vi "ConvertPB_AOupdates.vi"(0 "PB VLIW Array in":T2(array[cluster]) {"Output Bits" format="%x"}, 1 "Definitions":T1={"External MemorySize"=32768, "Internal Memory Size"=512, "Overhead Ticks"=3, "Min Delay Loops"=3, "Loop Count Correction"=1, "Long Delay Loop Count Correction"=2, "Min Instruction Ticks"=6, "Long Delay Ticks"=4294967295, "Clock Period (s)"=1e-08, "Overhead Time (s)"=3e-08, "Min Instruction Cycle Time (s)"=9e-08, "Long Delay Time (s) "=42.94967298} {"Long Delay Time (s)" format="%.8p"; "Min Instruction Cycle Time (s)" format="%.0p"; "Overhead Time (s)" format="%.0p"; "Clock Period (s)" format="%.0p"; "Long Delay Ticks" format="%.0x"}, 2 "error in (no error)":errorcluster, 3 "Full trigger mask":u32 format="%x") -> (5 "PB VLIW Array out":T2(array[cluster]) {"Output Bits" format="%x"}, 6 "error out":errorcluster)   [LabVIEW 2013, in "PulseBlaster.lvlib"]
doc: "Convert AO updates to two pulses to allow consecutive AO pulses. Replicates the whole PB sequence execpt for channel 22 (AO tigger) and the PB halt channel."
uses:
  PulseBlaster.lvlib
panel:
  # "(Period*Long D Ticks)+Overhead time"
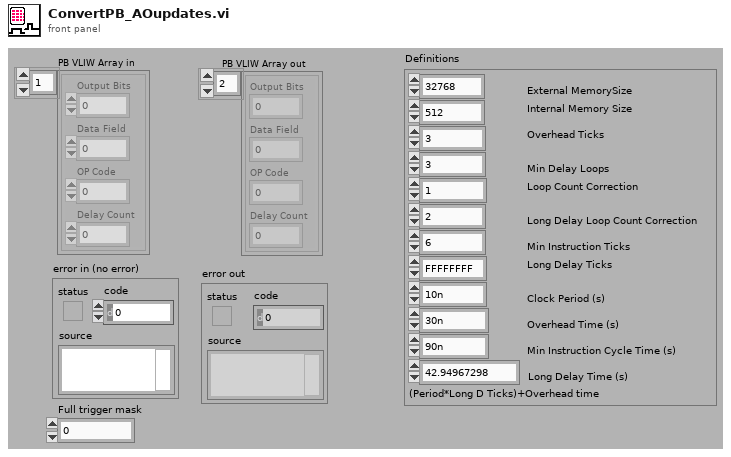
[diagram p1: front panel]
types:
  T1 = cluster{"External MemorySize":u16, "Internal Memory Size":u16, "Overhead Ticks":u8, "Min Delay Loops":u8, "Loop Count Correction":u8, "Long Delay Loop Count Correction":u8, "Min Instruction Ticks":u8, "Long Delay Ticks":u64, "Clock Period (s)":dbl, "Overhead Time (s)":dbl, "Min Instruction Cycle Time (s)":dbl, "Long Delay Time (s) ":dbl}
  T2 = cluster{"Output Bits":u32, "Data Field":u32, "OP Code":u8, "Delay Count":u64}[]
  T3 = cluster{"Output Bits":u32, "Data Field":u32, "OP Code":u8, "Delay Count":u32}[]
  T4 = cluster{"Output Bits":u32, "Data Field":u32, "OP Code":u8, "Delay Count":u64}
  T5 = cluster{"Output Bits":u32, "Data Field":u32, "OP Code":i32, "Delay Count":u64}[]
  T6 = cluster{"Output Bits":u32, "Data Field":u32, "OP Code":u8, u64}
  T7 = cluster{"Output Bits":u32, u32, "OP Code":u8, "Delay Count":u64}
  T8 = cluster{"Output Bits":u32, "Data Field":u32, i32, u64}
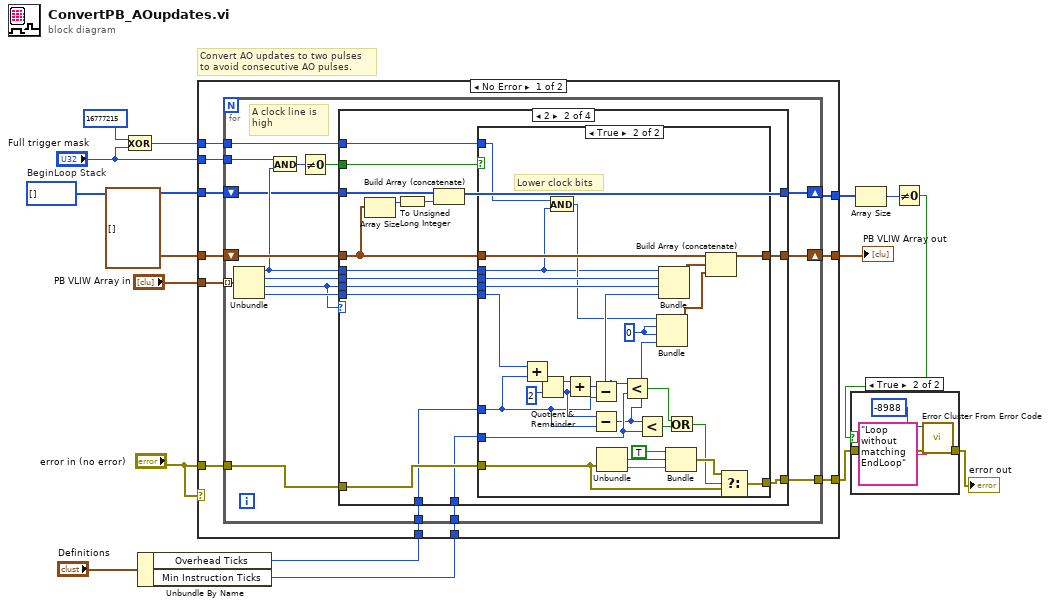
[diagram p0: block diagram]
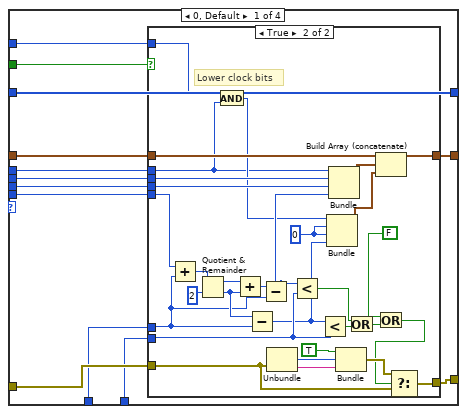
[diagram p3: hidden frame]
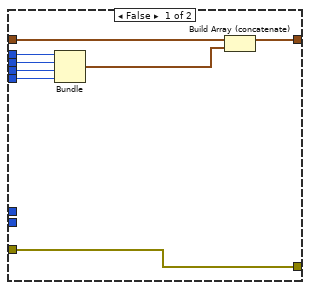
[diagram p4: hidden frame]
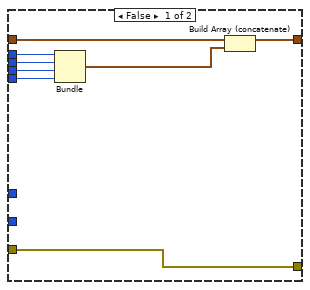
[diagram p5: hidden frame]
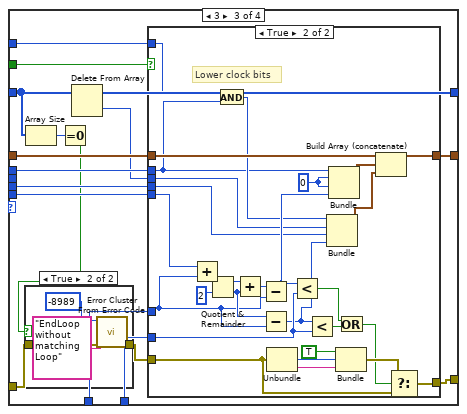
[diagram p6: hidden frame]
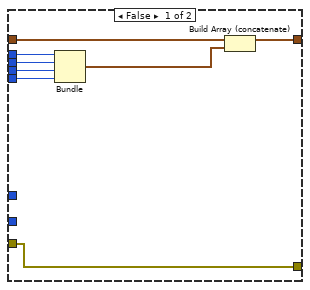
[diagram p8: hidden frame]
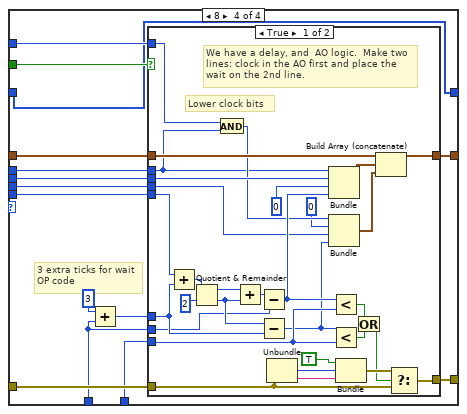
[diagram p9: hidden frame]
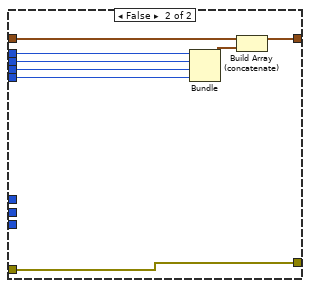
[diagram p10: hidden frame]
diagram:
  w6 = u32[] []  # BeginLoop Stack
  # "Convert AO updates to two pulses\nto avoid consecutive AO pulses."
  n1 = Exclusive Or(1:"Full trigger mask", 2:u32 16777215) -> (0:w10:u32)
  n2 = Unbundle By Name("Definitions") -> ("Overhead Ticks"=w8:u8, "Min Instruction Ticks"=w7:u8)
  n3 = case shown="No Error" "error in (no error)" {
    tunnel: T3 [] -> [w27 _]
    tunnel: [w26 w265] -> w15
    tunnel: w8 -> [w25 _]
    tunnel: w7 -> [w24 _]
    tunnel: "PB VLIW Array in" -> [w23 w265]
    tunnel: "error in (no error)" -> [w22 w264]
    tunnel: [w21 w264] -> w4
    tunnel: "Full trigger mask" -> [w20 _]
    tunnel: w10 -> [w19 _]
    tunnel: w6 -> [w18 w263]
    tunnel: [w17 w263] -> w3
    frame No Error {
      n4 = for {
        tunnel: w23 -> [w44] mode=indexing
        shift-right: [w36] -> w26
        shift-left: w27 -> [w41]
        tunnel: w22 -> [w40]
        tunnel: [w39] -> w21
        tunnel: w25 -> [w38]
        tunnel: w24 -> [w37]
        tunnel: w20 -> [w31]
        tunnel: w19 -> [w30]
        shift-right: [w29] -> w17
        shift-left: w18 -> [w28]
        # "A clock line is \nhigh"
        n5 = Unbundle(w44) -> ("Output Bits"=w34:u32, "Data Field"=w43:u32, "OP Code"=w35:u8, "Delay Count"=w42:u64)
        n6 = And(x=w31, y=w34) -> (x .and. y?=w33:u32)
        n7 = Not Equal To 0?(x=w33) -> (x != 0?=w32:bool)
        n8 = case shown="2" w35 {
          tunnel: w43 -> [w57 w112 _ w223]
          tunnel: w35 -> [w56 w111 w166 w222]
          tunnel: w42 -> [w55 w110 w165 w221]
          tunnel: w41 -> [w54 w103 w159 w220]
          tunnel: w40 -> [w53 w109 w151 w219]
          tunnel: [w52 w108 w164 w218] -> w39
          tunnel: w38 -> [w51 w107 w163 w211]
          tunnel: w37 -> [w50 w106 w162 w217]
          tunnel: w34 -> [w49 w105 w161 w216]
          tunnel: [w48 w104 w160 w215] -> w36
          tunnel: w32 -> [w47 w102 w158 w214]
          tunnel: w30 -> [w46 w101 w157 w210]
          tunnel: [w45 w99 w156 w209] -> w29
          tunnel: w28 -> [w45 w98 w154 w209]
          frame 0, Default {
            n9 = case shown="True" w47 {
              tunnel: w49 -> [w65 w67]
              tunnel: w57 -> [w64 w86]
              tunnel: w56 -> [w63 w75]
              tunnel: w55 -> [w62 w96]
              tunnel: [w60 w89] -> w48
              tunnel: w54 -> [w59 w88]
              tunnel: [w58 w81] -> w52
              tunnel: w53 -> [w58 w80]
              tunnel: w51 -> [_ w79]
              tunnel: w50 -> [_ w78]
              tunnel: w46 -> [_ w66]
              frame False {
                n10 = Bundle("Output Bits"=w65, "Data Field"=w64, "OP Code"=w63, "Delay Count"=w62) -> (w61:T4)  [unwired: 1 out]
                n11 = Build Array (concatenate)(w59, w61) -> (w60:T5)
              }
              frame True {
                w68 = 0
                # "Lower clock bits"
                n12 = Add(x=w96, y=w79) -> (x+y=w95:u64)
                n13 = Quotient & Remainder(x=w95, y=u32 2) -> (x-y*floor(x/y)=w93:u64, floor(x/y)=w91:u64)
                n14 = And(x=w66, y=w67) -> (x .and. y?=w74:u32)
                n15 = Add(x=w93, y=w91) -> (x+y=w92:u64)
                n16 = Subtract(x=w91, y=w79) -> (x-y=w76:u64)
                n17 = Subtract(x=w92, y=w79) -> (x-y=w87:u64)
                n18 = Unbundle(w80) -> ("code"=w83:i32, "source"=w84:string)  [unwired: 1 out]
                n19 = Less?(x=w87, y=w78) -> (x < y?=w90:bool)
                n20 = Less?(x=w76, y=w78) -> (x < y?=w77:bool)
                n21 = Bundle(w74, w68, w68, w76) -> (w69:cluster{u32, i32, i32, u64})  [unwired: 1 out]
                n22 = Bundle("Output Bits"=w67, "Data Field"=w86, "OP Code"=w75, w87) -> (w70:T6)  [unwired: 1 out]
                n23 = Bundle(TRUE, "code"=w83, "source"=w84) -> (w82:cluster{bool, "code":i32, "source":string})  [unwired: 1 out]
                n24 = Or(x=w90, y=w77) -> (x .or. y?=w71:bool)
                n25 = Build Array (concatenate)(w88, w70, w69) -> (w89:T5)
                n26 = Or(x=FALSE, y=w71) -> (x .or. y?=w72:bool)
                n27 = Select(t=w82, s=w72, f=w80) -> (s? t:f=w81:errorcluster)
              }
            }
          }
          frame 2 {
            n28 = Array Size(array=w103) -> (size(s)=w97:i32)
            n29 = To Unsigned Long Integer(number=w97) -> (unsigned 32bit integer=w100:u32)
            n30 = Build Array (concatenate)(w98, w100) -> (w99:u32[])
            n31 = case shown="True" w102 {
              tunnel: w105 -> [w120 w122]
              tunnel: w112 -> [w119 w139]
              tunnel: w111 -> [w118 w128]
              tunnel: w110 -> [w117 w149]
              tunnel: [w115 w142] -> w104
              tunnel: w103 -> [w114 w141]
              tunnel: [w113 w134] -> w108
              tunnel: w109 -> [w113 w133]
              tunnel: w107 -> [_ w132]
              tunnel: w106 -> [_ w131]
              tunnel: w101 -> [_ w121]
              frame False {
                n32 = Bundle("Output Bits"=w120, "Data Field"=w119, "OP Code"=w118, "Delay Count"=w117) -> (w116:T4)  [unwired: 1 out]
                n33 = Build Array (concatenate)(w114, w116) -> (w115:T5)
              }
              frame True {
                w124 = 0
                # "Lower clock bits"
                n34 = Add(x=w149, y=w132) -> (x+y=w148:u64)
                n35 = Quotient & Remainder(x=w148, y=u32 2) -> (x-y*floor(x/y)=w146:u64, floor(x/y)=w144:u64)
                n36 = And(x=w121, y=w122) -> (x .and. y?=w127:u32)
                n37 = Add(x=w146, y=w144) -> (x+y=w145:u64)
                n38 = Subtract(x=w145, y=w132) -> (x-y=w140:u64)
                n39 = Subtract(x=w144, y=w132) -> (x-y=w129:u64)
                n40 = Unbundle(w133) -> ("code"=w136:i32, "source"=w137:string)  [unwired: 1 out]
                n41 = Less?(x=w140, y=w131) -> (x < y?=w143:bool)
                n42 = Less?(x=w129, y=w131) -> (x < y?=w130:bool)
                n43 = Bundle(w127, w124, w124, w129) -> (w125:cluster{u32, i32, i32, u64})  [unwired: 1 out]
                n44 = Bundle("Output Bits"=w122, "Data Field"=w139, "OP Code"=w128, w140) -> (w126:T6)  [unwired: 1 out]
                n45 = Bundle(TRUE, "code"=w136, "source"=w137) -> (w135:cluster{bool, "code":i32, "source":string})  [unwired: 1 out]
                n46 = Or(x=w143, y=w130) -> (x .or. y?=w123:bool)
                n47 = Build Array (concatenate)(w141, w126, w125) -> (w142:T5)
                n48 = Select(t=w135, s=w123, f=w133) -> (s? t:f=w134:errorcluster)
              }
            }
          }
          frame 3 {
            n49 = Array Size(array=w154) -> (size(s)=w153:i32)
            n50 = Equal To 0?(x=w153) -> (x = 0?=w152:bool)
            n51 = case shown="True" w152 {
              tunnel: w151 -> [w167 w169]
              tunnel: [w167 w168] -> w150
              frame False {
              }
              frame True {
                n52 = call <vilib>:"Error Cluster From Error Code.vi"("error in (no error)"=w169, "error message (\"\")"="EndLoop without matching Loop" ("error message (\"\")"), "error code (0)"=-8989) -> ("error out"=w168:errorcluster)  [unwired: 6 in]
              }
            }
            n53 = Delete From Array(array=w154) -> (deleted portion=w155:u32, array with subset deleted=w156:u32[])  [unwired: 2 in]
            n54 = case shown="True" w158 {
              tunnel: w161 -> [w179 w182]
              tunnel: w155 -> [w178 w198]
              tunnel: w166 -> [w177 w188]
              tunnel: w165 -> [w176 w208]
              tunnel: [w174 w201] -> w160
              tunnel: w159 -> [w173 w200]
              tunnel: [w172 w193] -> w164
              tunnel: w163 -> [_ w192]
              tunnel: w162 -> [_ w191]
              tunnel: w157 -> [_ w181]
              tunnel: w150 -> [w172 w180]
              frame False {
                n55 = Bundle("Output Bits"=w179, w178, "OP Code"=w177, "Delay Count"=w176) -> (w175:T7)  [unwired: 1 out]
                n56 = Build Array (concatenate)(w173, w175) -> (w174:T5)
              }
              frame True {
                w184 = 0
                # "Lower clock bits"
                n57 = Add(x=w208, y=w192) -> (x+y=w207:u64)
                n58 = Quotient & Remainder(x=w207, y=u32 2) -> (x-y*floor(x/y)=w205:u64, floor(x/y)=w203:u64)
                n59 = And(x=w181, y=w182) -> (x .and. y?=w187:u32)
                n60 = Add(x=w205, y=w203) -> (x+y=w204:u64)
                n61 = Subtract(x=w204, y=w192) -> (x-y=w199:u64)
                n62 = Subtract(x=w203, y=w192) -> (x-y=w189:u64)
                n63 = Unbundle(w180) -> ("code"=w195:i32, "source"=w196:string)  [unwired: 1 out]
                n64 = Less?(x=w199, y=w191) -> (x < y?=w202:bool)
                n65 = Less?(x=w189, y=w191) -> (x < y?=w190:bool)
                n66 = Bundle(w187, w198, "OP Code"=w188, w189) -> (w185:cluster{u32, u32, "OP Code":u8, u64})  [unwired: 1 out]
                n67 = Bundle("Output Bits"=w182, w184, w184, w199) -> (w186:cluster{"Output Bits":u32, i32, i32, u64})  [unwired: 1 out]
                n68 = Bundle(TRUE, "code"=w195, "source"=w196) -> (w194:cluster{bool, "code":i32, "source":string})  [unwired: 1 out]
                n69 = Or(x=w202, y=w190) -> (x .or. y?=w183:bool)
                n70 = Build Array (concatenate)(w200, w186, w185) -> (w201:T5)
                n71 = Select(t=w194, s=w183, f=w180) -> (s? t:f=w193:errorcluster)
              }
            }
          }
          frame 8 {
            # "3 extra ticks for wait\nOP code"
            n72 = Add(x=u8 3, y=w211) -> (x+y=w212:u8)
            n73 = case shown="True" w214 {
              tunnel: w216 -> [w225 w257]
              tunnel: w223 -> [w244 w260]
              tunnel: w222 -> [w228 w259]
              tunnel: w221 -> [w254 w256]
              tunnel: [w247 w262] -> w215
              tunnel: w220 -> [w246 w261]
              tunnel: [w239 w255] -> w218
              tunnel: w219 -> [w238 w255]
              tunnel: w212 -> [w237 _]
              tunnel: w217 -> [w236 _]
              tunnel: w211 -> [w226 _]
              tunnel: w210 -> [w224 _]
              frame True {
                # "We have a delay, and  AO logic.  Make two  lines: clock in the AO first and place the wait on the 2nd line."
                # "Lower clock bits"
                n74 = Add(x=w254, y=w237) -> (x+y=w253:u64)
                n75 = Quotient & Remainder(x=w253, y=u32 2) -> (x-y*floor(x/y)=w251:u64, floor(x/y)=w249:u64)
                n76 = And(x=w224, y=w225) -> (x .and. y?=w233:u32)
                n77 = Add(x=w251, y=w249) -> (x+y=w250:u64)
                n78 = Subtract(x=w250, y=w226) -> (x-y=w245:u64)
                n79 = Subtract(x=w249, y=w237) -> (x-y=w234:u64)
                n80 = Unbundle(w238) -> ("code"=w241:i32, "source"=w242:string)  [unwired: 1 out]
                n81 = Bundle("Output Bits"=w225, "Data Field"=w244, 0, w245) -> (w232:T8)  [unwired: 1 out]
                n82 = Bundle(w233, 0, "OP Code"=w228, w234) -> (w231:cluster{u32, i32, "OP Code":u8, u64})  [unwired: 1 out]
                n83 = Less?(x=w245, y=w236) -> (x < y?=w248:bool)
                n84 = Less?(x=w234, y=w236) -> (x < y?=w235:bool)
                n85 = Bundle(TRUE, "code"=w241, "source"=w242) -> (w240:cluster{bool, "code":i32, "source":string})  [unwired: 1 out]
                n86 = Or(x=w248, y=w235) -> (x .or. y?=w227:bool)
                n87 = Build Array (concatenate)(w246, w232, w231) -> (w247:T5)
                n88 = Select(t=w240, s=w227, f=w238) -> (s? t:f=w239:errorcluster)
              }
              frame False {
                n89 = Bundle("Output Bits"=w257, "Data Field"=w260, "OP Code"=w259, "Delay Count"=w256) -> (w258:T4)  [unwired: 1 out]
                n90 = Build Array (concatenate)(w261, w258) -> (w262:T5)
              }
            }
          }
        }
      }
    }
    frame Error {
    }
  }
  "PB VLIW Array out" <- w15
  n91 = Array Size(array=w3) -> (size(s)=w2:i32)
  n92 = Not Equal To 0?(x=w2) -> (x != 0?=w1:bool)
  n93 = case shown="True" w1 {
    tunnel: w4 -> [w266 w268]
    tunnel: [w266 w267] -> w5
    frame False {
    }
    frame True {
      n94 = call <vilib>:"Error Cluster From Error Code.vi"("error in (no error)"=w268, "error message (\"\")"="Loop without matching EndLoop" ("error message (\"\")"), "error code (0)"=-8988) -> ("error out"=w267:errorcluster)  [unwired: 6 in]
    }
  }
  "error out" <- w5
